vi "Increment Time (nanoseconds).vi"(8 "error in (no error)":errorcluster, 10 "nanos offset":i64, 11 "nanoseconds in":i64) -> (0 "error out":errorcluster, 3 "nanoseconds out":i64)   [LabVIEW 2013, in "Linux RT Utilities.lvlib"]
doc: "This VI increments the provided timespec by a number of nanoseconds."
uses:
  Linux RT Utilities.lvlib
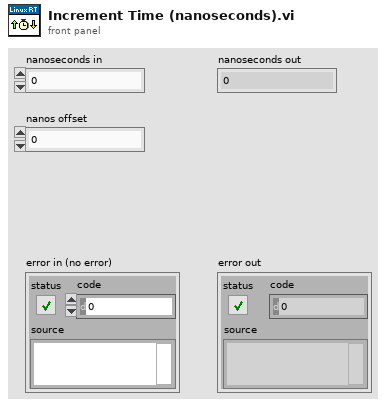
[diagram p1: front panel]
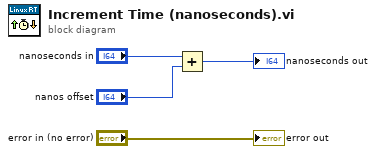
[diagram p0: block diagram]
diagram:
  n1 = Add(x="nanoseconds in", y="nanos offset") -> (x+y=→"nanoseconds out":i64)
  "error out" <- "error in (no error)"
